vi "Switch Logic Analyzer State.vi"(8 "error in (no error)":errorcluster, 11 "VISA resource name":refnum<visa-resource-name>) -> (0 "error out":errorcluster, 3 "VISA resource name out":refnum<visa-resource-name>)   [LabVIEW 2012, in "RIGOL DS1000 Series.lvlib"]
doc: "Enables or disables the logic analyzer built-in the oscilloscope.The On/Off state of the analyzer switched once you call this VI continuously.\n\nNote:\nThis VI is only valid for DS1052D and DS1102D."
uses:
  RIGOL DS1000 Series.lvlib
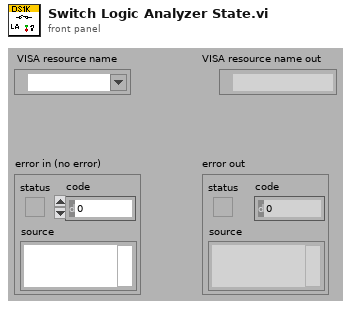
[diagram p1: front panel]
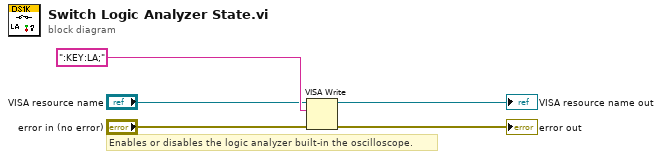
[diagram p0: block diagram]
diagram:
  # "Enables or disables the logic analyzer built-in the oscilloscope."
  n1 = VISA Write(VISA resource name="VISA resource name", write buffer=":KEY:LA;", error in (no error)="error in (no error)") -> (VISA resource name out=→"VISA resource name out":refnum<visa-resource-name>, error out=→"error out":errorcluster)  [unwired: 1 out]
